vi "Init.vi"(8 "error in (no error)":errorcluster, 11 "Port Selection Info In":T1={"Port Name"="", "Amplifier Num"=1, "Baud Rate"=38400, "Char Formation"=enum."0"} {"Baud Rate" items=["38400"=38400, "19200"=19200, "9600"=9600, "115200"=0]; "Amplifier Num" max=31}) -> (0 "error out":errorcluster, 3 "Fuji Delta out":refnum<class "Fuji Delta Robot.lvclass">)   [LabVIEW 2014, in "Fuji Delta Robot.lvlib" / "Fuji Delta Robot.lvclass"]
uses:
  Fuji Delta Robot.lvclass
  ALPHA5 RS485/typedefs/Port Selection Info.ctl
  Fuji Delta Robot.lvclass/Fuji Delta Robot.ctl
  ALPHA5 RS485/Classes/FujiMotor/FujiMotor.lvclass
  ALPHA5 RS485/ALPHA5 RS485.lvlib
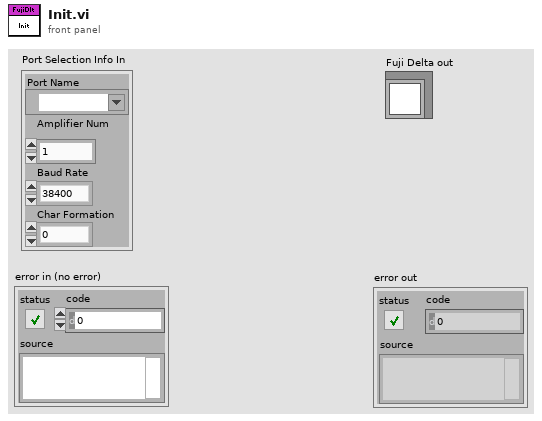
[diagram p1: front panel]
types:
  T1 = typedef "ALPHA5 RS485.lvlib/Port Selection Info.ctl" = cluster{"Port Name":refnum<visa-resource-name>, "Amplifier Num":u8, "Baud Rate":u32, "Char Formation":enum16{"0", "1", "2", "3", "4", "5"}}
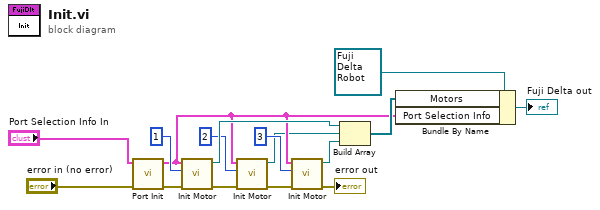
[diagram p0: block diagram]
diagram:
  n1 = call "Port Init.vi"("error in (no error)"="error in (no error)", "Port Selection Info In"="Port Selection Info In") -> ("error out"=w9:errorcluster, "Port Selection Info Out"=w5:T1)  [unwired: 8 in]
  n2 = call "Init Motor.vi"("error in (no error)"=w9, "Motor ID"=u8 1, "Port Selection Info In"=w5) -> ("error out"=w8:errorcluster, "FujiMotor out"=w13:refnum<class "FujiMotor.lvclass">)  [unwired: 7 in]
  n3 = call "Init Motor.vi"("error in (no error)"=w8, "Motor ID"=u8 2, "Port Selection Info In"=w5) -> ("error out"=w6:errorcluster, "FujiMotor out"=w3:refnum<class "FujiMotor.lvclass">)  [unwired: 7 in]
  n4 = call "Init Motor.vi"("error in (no error)"=w6, "Motor ID"=u8 3, "Port Selection Info In"=w5) -> ("error out"=→"error out":errorcluster, "FujiMotor out"=w2:refnum<class "FujiMotor.lvclass">)  [unwired: 7 in]
  n5 = Build Array(w13, w3, w2) -> (w14:refnum<class "FujiMotor.lvclass">[])
  n6 = Bundle By Name(cluster=refnum<class "Fuji Delta Robot.lvclass"> refnum ("Fuji Delta Robot.lvlib:Fuji Delta Robot.lvclass"), "Motors"=w14, "Port Selection Info"=w5) -> (→"Fuji Delta out":refnum<class "Fuji Delta Robot.lvclass">)
